vi "io.frame.vi"(8 "error in":errorcluster, 9 "Direction (To RIO)":enum16{"SendToRIO", "ReceiveFromRio"}(ring), 10 "Frameless Command":string) -> (0 "error out":errorcluster, 2 "Framed Command":string)   [LabVIEW 2024]
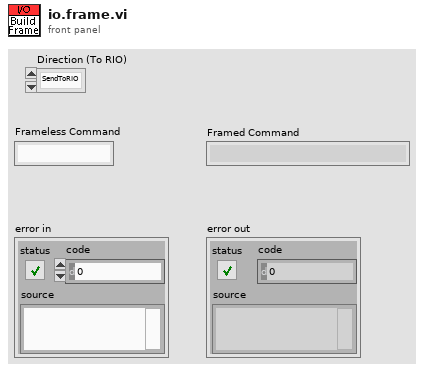
[diagram p1: front panel]
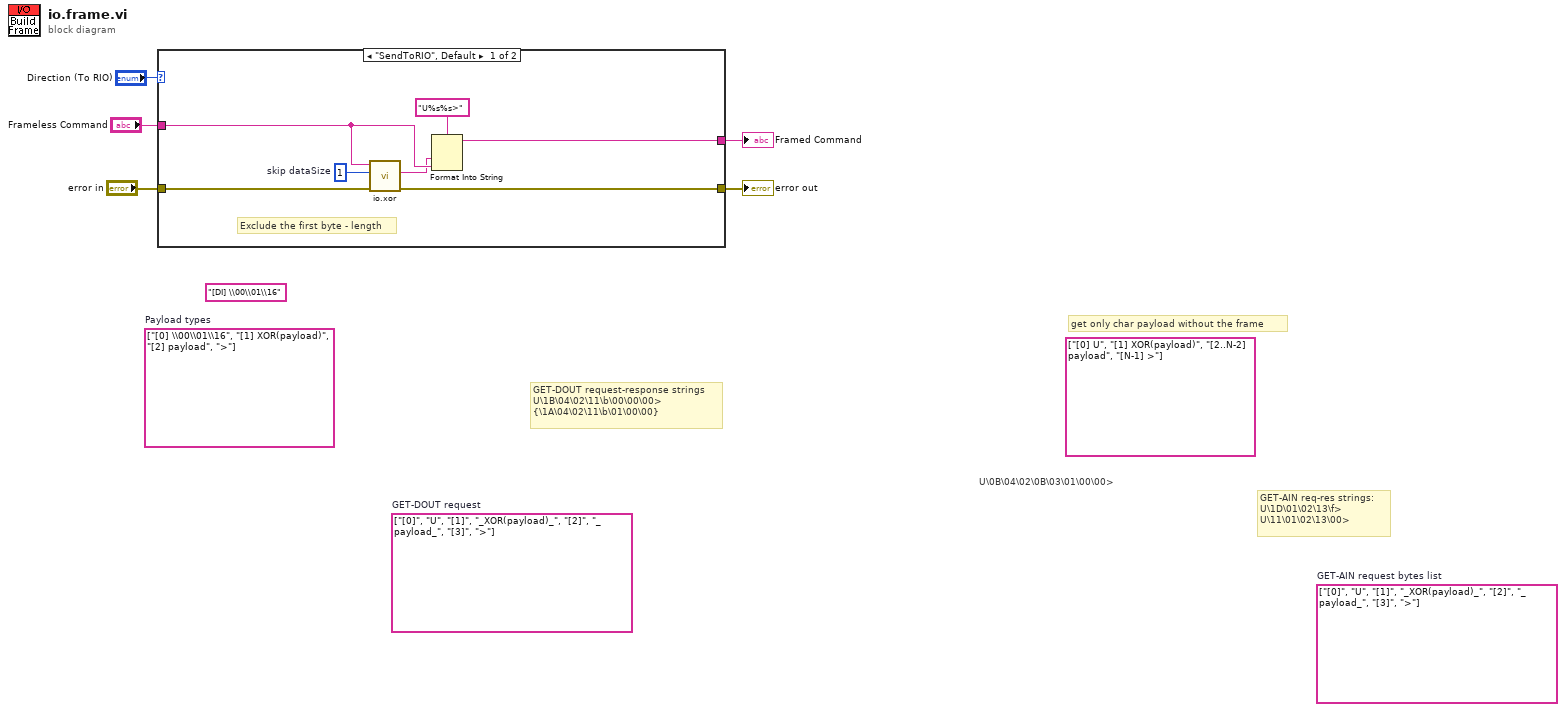
[diagram p0: block diagram]
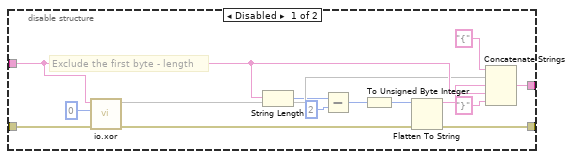
[diagram p3: hidden frame]
diagram:
  (unwired) "[DI] \\00\\01\\16" ("String")
  (unwired) string[][] [["[0]", "U"], ["[1]", "_XOR(payload)_"], ["[2]", "_payload_"], ["[3]", ">"]]  # GET-AIN request bytes list
  (unwired) string[][] [["[0]", "U"], ["[1]", "_XOR(payload)_"], ["[2]", "_payload_"], ["[3]", ">"]]  # GET-DOUT request
  (unwired) string[] ["[0] \\00\\01\\16", "[1] XOR(payload)", "[2] payload", ">"]  # Payload types
  (unwired) string[] ["[0] U", "[1] XOR(payload)", "[2..N-2] payload", "[N-1] >"]
  # "GET-AIN req-res strings: \nU\\1D\\01\\02\\13\\f>\nU\\11\\01\\02\\13\\00>"
  # "GET-DOUT request-response strings\nU\\1B\\04\\02\\11\\b\\00\\00\\00>\n{\\1A\\04\\02\\11\\b\\01\\00\\00}"
  # "U\\0B\\04\\02\\0B\\03\\01\\00\\00>"
  # "get only char payload without the frame"
  n1 = case shown="\"SendToRIO\", Default" "Direction (To RIO)" {
    tunnel: [w6 w16] -> w5
    tunnel: [w12 w15] -> w4
    tunnel: "Frameless Command" -> [w8 w14]
    tunnel: "error in" -> [w10 w13]
    frame "SendToRIO", Default {
      w11 = u8 1  # skip dataSize
      # "Exclude the first byte - length"
      n2 = call "io.xor.vi"("error in"=w10, "Start Index (0)"=w11, "payload in"=w8) -> ("error out"=w12:errorcluster, "XOR(payload)"=w7:string)  [unwired: 6 in, 1 out]
      n3 = Format Into String(format string="U%s%s>" ("string"), w7, w8) -> (resulting string=w6:string)  [unwired: 2 in, 1 out]
    }
    frame "ReceiveFromRio" {
      n4 = disable-structure shown="Enabled" {
        disable-tunnel: [w30 _] -> w16
        disable-tunnel: [w29 _] -> w15
        disable-tunnel: w14 -> [w28 _]
        disable-tunnel: w13 -> [w24 _]
        frame Disabled {
          # "Exclude the first byte - length"
          n5 = call "io.xor.vi"("error in"=w24, "Start Index (0)"=u8 0, "payload in"=w28) -> ("error out"=w25:errorcluster, 3:w26)  [unwired: 5 in, 2 out]
          n6 = String Length(string=w28) -> (length=w19:i32)
          n7 = Subtract(x=w19, y=2) -> (x-y=w18:i32)
          n8 = To Unsigned Byte Integer(number=w18) -> (unsigned 8bit integer=w21:u8)
          n9 = Flatten To String(anything=w21, error in (no error)=w25) -> (data string=w20:string, error out=w29:errorcluster)  [unwired: 2 in, 1 out]
          n10 = Concatenate Strings("{" ("string"), w26, w20, w28, "}" ("string")) -> (w30:string)
        }
        frame Enabled {
        }
      }
    }
  }
  "Framed Command" <- w5
  "error out" <- w4
